vi "AssembleVelocityStats.vi"(7 "TitlePrefix":string, 11 "VmagUVWCone":dbl[][](array[numeric])) -> (1 "Plug in titles":string[](array[string]), 3 "StatsArray":dbl[](array[numeric]))   [LabVIEW 2013]
uses:
  <vilib>/Analysis/NI_AALBase.lvlib
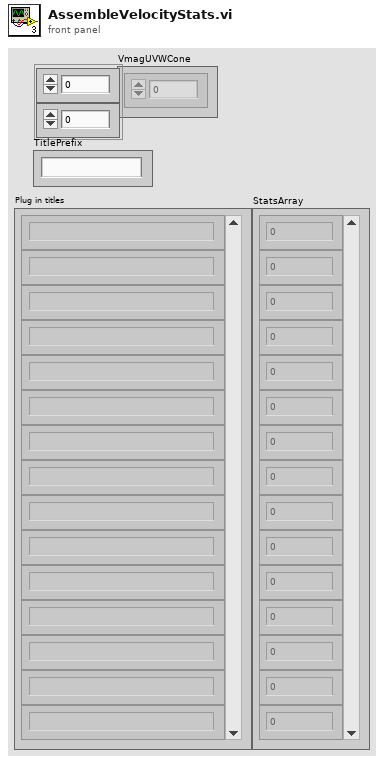
[diagram p1: front panel]
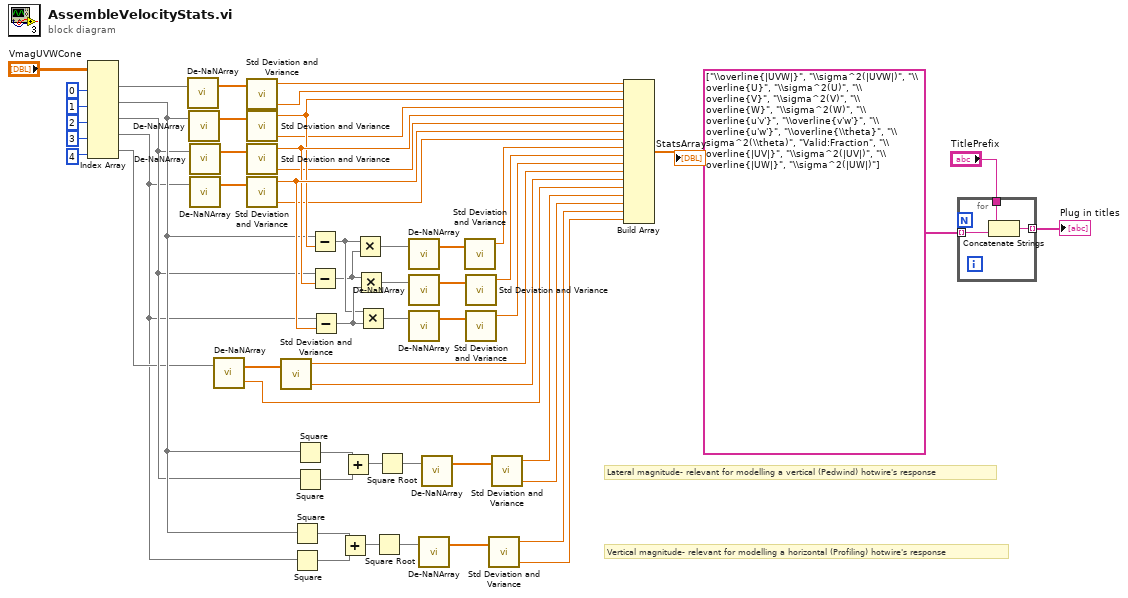
[diagram p0: block diagram]
diagram:
  # "Vertical magnitude- relevant for modelling a horizontal (Profiling) hotwire's response"
  # "Lateral magnitude- relevant for modelling a vertical (Pedwind) hotwire's response"
  n1 = Index Array(array="VmagUVWCone", index (col) #1=0 ("disabled index (col)"), index (col) #2=1 ("index (col)"), index (col) #3=2 ("index (col)"), index (col) #4=3 ("index (col)"), index (col) #5=4 ("index (col)")) -> (element #1=w6:dbl[], element #2=w4:dbl[], element #3=w3:dbl[], element #4=w1:dbl[], element #5=w2:dbl[])  [unwired: 5 in]
  n2 = call "De-NaNArray.vi"("ArrayIn"=w6) -> ("de-NaN-dArrayOut"=w21:dbl[])  [unwired: 1 in, 1 out]
  n3 = call "De-NaNArray.vi"("ArrayIn"=w4) -> ("de-NaN-dArrayOut"=w30:dbl[])  [unwired: 1 in, 1 out]
  n4 = call "De-NaNArray.vi"("ArrayIn"=w3) -> ("de-NaN-dArrayOut"=w29:dbl[])  [unwired: 1 in, 1 out]
  n5 = call "De-NaNArray.vi"("ArrayIn"=w1) -> ("de-NaN-dArrayOut"=w28:dbl[])  [unwired: 1 in, 1 out]
  n6 = call "De-NaNArray.vi"("ArrayIn"=w2) -> ("GoodFraction"=w20:dbl, "de-NaN-dArrayOut"=w31:dbl[])  [unwired: 1 in]
  n7 = call <vilib>:"Std Deviation and Variance.vi"("X"=w21) -> ("mean"=w45:dbl, "variance"=w40:dbl)  [unwired: 1 in, 1 out]
  n8 = call <vilib>:"Std Deviation and Variance.vi"("X"=w30) -> ("mean"=w46:dbl, "variance"=w41:dbl)  [unwired: 1 in, 1 out]
  n9 = call <vilib>:"Std Deviation and Variance.vi"("X"=w29) -> ("mean"=w47:dbl, "variance"=w42:dbl)  [unwired: 1 in, 1 out]
  n10 = call <vilib>:"Std Deviation and Variance.vi"("X"=w28) -> ("mean"=w48:dbl, "variance"=w43:dbl)  [unwired: 1 in, 1 out]
  n11 = call <vilib>:"Std Deviation and Variance.vi"("X"=w31) -> ("mean"=w56:dbl, "variance"=w57:dbl)  [unwired: 1 in, 1 out]
  n12 = Square(x=w4) -> (x^2=w9:dbl[])
  n13 = Square(x=w1) -> (x^2=w10:dbl[])
  n14 = Square(x=w4) -> (x^2=w19:dbl[])
  n15 = Square(x=w3) -> (x^2=w18:dbl[])
  n16 = Subtract(x=w4, y=w46) -> (x-y=w50:dbl[])
  n17 = Subtract(x=w3, y=w47) -> (x-y=w49:dbl[])
  n18 = Subtract(x=w1, y=w48) -> (x-y=w51:dbl[])
  n19 = Add(x=w9, y=w10) -> (x+y=w11:dbl[])
  n20 = Add(x=w19, y=w18) -> (x+y=w17:dbl[])
  n21 = Multiply(x=w50, y=w49) -> (x*y=w27:dbl[])
  n22 = Multiply(x=w49, y=w51) -> (x*y=w25:dbl[])
  n23 = Multiply(x=w50, y=w51) -> (x*y=w23:dbl[])
  n24 = Square Root(x=w11) -> (sqrt(x)=w12:dbl[])
  n25 = Square Root(x=w17) -> (sqrt(x)=w5:dbl[])
  n26 = call "De-NaNArray.vi"("ArrayIn"=w27) -> ("de-NaN-dArrayOut"=w26:dbl[])  [unwired: 1 in, 1 out]
  n27 = call "De-NaNArray.vi"("ArrayIn"=w25) -> ("de-NaN-dArrayOut"=w24:dbl[])  [unwired: 1 in, 1 out]
  n28 = call "De-NaNArray.vi"("ArrayIn"=w23) -> ("de-NaN-dArrayOut"=w22:dbl[])  [unwired: 1 in, 1 out]
  n29 = call "De-NaNArray.vi"("ArrayIn"=w12) -> ("de-NaN-dArrayOut"=w13:dbl[])  [unwired: 1 in, 1 out]
  n30 = call "De-NaNArray.vi"("ArrayIn"=w5) -> ("de-NaN-dArrayOut"=w16:dbl[])  [unwired: 1 in, 1 out]
  n31 = call <vilib>:"Std Deviation and Variance.vi"("X"=w26) -> ("mean"=w52:dbl)  [unwired: 1 in, 2 out]
  n32 = call <vilib>:"Std Deviation and Variance.vi"("X"=w24) -> ("mean"=w53:dbl)  [unwired: 1 in, 2 out]
  n33 = call <vilib>:"Std Deviation and Variance.vi"("X"=w22) -> ("mean"=w54:dbl)  [unwired: 1 in, 2 out]
  n34 = call <vilib>:"Std Deviation and Variance.vi"("X"=w13) -> ("mean"=w8:dbl, "variance"=w7:dbl)  [unwired: 1 in, 1 out]
  n35 = call <vilib>:"Std Deviation and Variance.vi"("X"=w16) -> ("mean"=w15:dbl, "variance"=w14:dbl)  [unwired: 1 in, 1 out]
  n36 = Build Array(w45, w40, w46, w41, w47, w42, w48, w43, w52, w53, w54, w56, w57, w20, w15, w14, w8, w7) -> (→"StatsArray":dbl[])
  n37 = for {
    tunnel: string[] ["\\overline{|UVW|}", "\\sigma^2(|UVW|)", "\\overline{U}", "\\sigma^2(U)", "\\overline{V}", "\\sigma^2(V)", "\\overline{W}", "\\sigma^2(W)", "\\overline{u'v'}", "\\overline{v'w'}", "\\overline{u'w'}", "\\overline{\\theta}", "\\sigma^2(\\theta)", "Valid:Fraction", "\\overline{|UV|}", "\\sigma^2(|UV|)", "\\overline{|UW|}", "\\sigma^2(|UW|)"] ("Plug in titles") -> [w60] mode=indexing
    tunnel: "TitlePrefix" -> [w59]
    tunnel: [w58] -> w32 mode=indexing
    n38 = Concatenate Strings(w59, w60) -> (w58:string)
  }
  "Plug in titles" <- w32
